vi "sub_tabelle_anhaengen.vi"(0 "Beschreibung":string, 1 "Wellenlänge":string, 2 "Aktuelle xyz-Position [mm]":dbl[](array[numeric]) format="%.5g") -> ()   [LabVIEW 2009]
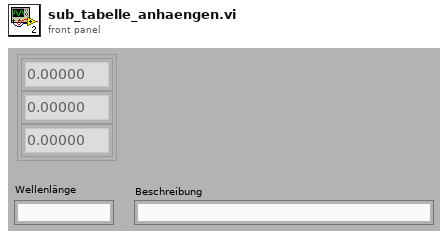
[diagram p1: front panel]
types:
  T1 = enum16{"open", "replace", "create", "open or create", "replace or create", "replace or create with confirmation"}
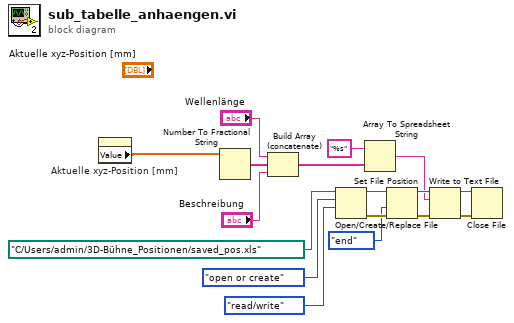
[diagram p0: block diagram]
diagram:
  n1 = property on="Aktuelle xyz-Position [mm]" class="Arr (strikt)"() -> ("Value"=w1:dbl[])  [unwired: 2 in, 2 out]
  n2 = Number To Fractional String(number=w1) -> (F-format string=w16:string[])  [unwired: 3 in]
  n3 = Build Array (concatenate)("Wellenlänge", w16, "Beschreibung") -> (w14:string[])
  n4 = Open/Create/Replace File(file path (use dialog)=path "C:/Users/admin/3D-Bühne_Positionen/saved_pos.xls" ("Dateipfad (Dialog verwenden)"), operation (0:open)=T1."open or create" ("Operation (0:Öffnen)"), access (0:read/write)=enum16{"read/write", "read-only", "write-only"}."read/write" ("Zugriff (0:Lesen/Schreiben)")) -> (refnum out=w8:refnum<file>, error out=w9:errorcluster)  [unwired: 3 in, 1 out]
  n5 = Array To Spreadsheet String(array=w14, 3:"%s" ("Format-String")) -> (spreadsheet string=w4:string)  [unwired: 1 in]
  n6 = Set File Position(refnum=w8, from (0:start)=enum16{"start", "end", "current"}."end" ("Von (0:Start)"), error in=w9) -> (refnum out=w6:refnum<file>, error out=w5:errorcluster)  [unwired: 1 in]
  n7 = Write to Text File(file (use dialog)=w6, text=w4, error in=w5) -> (refnum out=w2:refnum<file>, error out=w3:errorcluster)  [unwired: 1 in, 1 out]
  n8 = Close File(refnum=w2, error in=w3) -> ()  [unwired: 2 out]
